vi "GetOpMode.vi"(8 "error in (no error)":errorcluster, 11 "BME680 in":refnum<class "BME680.lvclass">) -> (0 "error out":errorcluster, 2 "Op Mode":u8, 3 "BME680 out":refnum<class "BME680.lvclass">)   [LabVIEW 2022 SP3, in "BME680.lvlib" / "BME680.lvclass"]
uses:
  BME680.lvclass
  BME680.lvclass/BME680.ctl
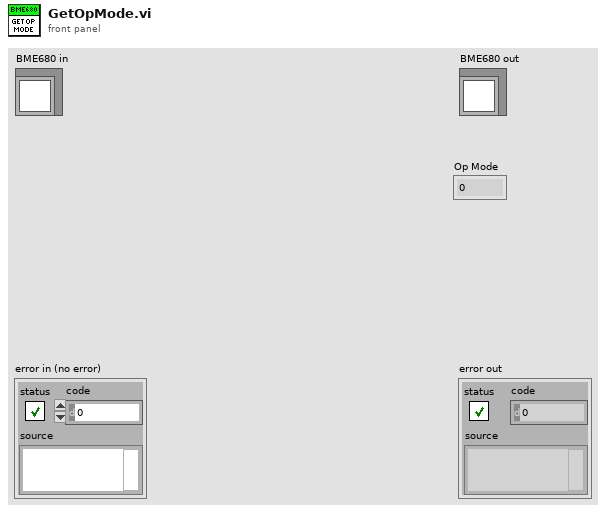
[diagram p1: front panel]
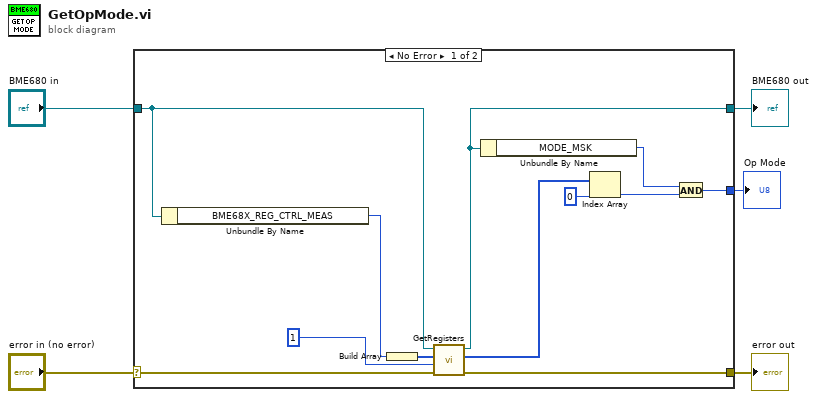
[diagram p0: block diagram]
diagram:
  n1 = case shown="No Error" "error in (no error)" {
    selector: "error in (no error)" -> [w17 w19]
    tunnel: [w16 w19] -> w4
    tunnel: [w9 w18] -> w2
    tunnel: "BME680 in" -> [w15 w18]
    tunnel: [w6 _] -> w1
    frame No Error {
      n2 = Unbundle By Name(w15) -> ("BME68X_REG_CTRL_MEAS"=w13:u8)
      n3 = Build Array(w13) -> (w14:u8[])
      n4 = call-dynamic "GetRegisters.vi"("error in (no error)"=w17, "Lenght"=u8 1, "Addr"=w14, "BME680 in"=w15) -> ("error out"=w16:errorcluster, "Data out"=w11:u8[], "BME680 out"=w9:refnum<class "BME680.lvclass">)  [unwired: 5 in]
      n5 = Unbundle By Name(w9) -> ("MODE_MSK"=w7:u8)
      n6 = Index Array(array=w11, index=0) -> (element=w8:u8)
      n7 = And(x=w7, y=w8) -> (x .and. y?=w6:u8)
    }
    frame Error {
    }
  }
  "error out" <- w4
  "BME680 out" <- w2
  "Op Mode" <- w1
